vi "主函数.vi"() -> ()   [LabVIEW 2018]
panel:
  out "数值":dbl
  in  "a":dbl
  in  "c":dbl
  in  "b":dbl
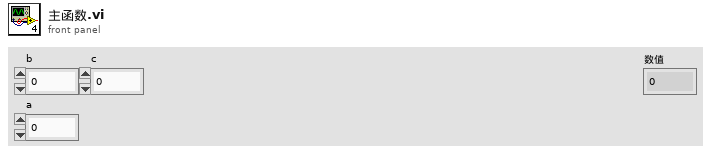
[diagram p1: front panel]
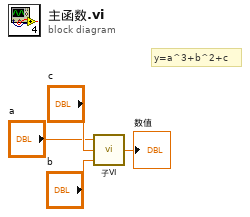
[diagram p0: block diagram]
diagram:
  # "y=a^3+b^2+c"
  n1 = call "子VI.vi"("b"="b", "c"="c", "a"="a") -> ("数值"=→"数值":dbl)
